vi "DriveModuleControl_TravTuneKa.vi"(8 "error in":errorcluster, 9 "Actual State":T1={"Speed"=0.0, "Angle"={"VALUE"=0.0, "COS"=1.0, "SIN"=0.0}} {"Angle"."SIN" format="%13.4f"; "Angle"."COS" format="%13.4f"; "Angle"."VALUE" format="%13.4f"}, 10 "Desired State":T1={"Speed"=0.0, "Angle"={"VALUE"=0.0, "COS"=1.0, "SIN"=0.0}} {"Angle"."SIN" format="%13.4f"; "Angle"."COS" format="%13.4f"; "Angle"."VALUE" format="%13.4f"}, 11 "ModualNamePrefix":i32) -> (0 "error out":errorcluster)   [LabVIEW 2023]
uses:
  <vilib>/Rock Robotics/WPI/ThirdParty/JAS_Junk/TrajLib/TypeDef/SWERVE_DRIVE_MODULE_STATE.ctl
  <vilib>/Rock Robotics/WPI/ThirdParty/JAS_Junk/TrajLib/TypeDef/ROTATION2D.ctl
  <vilib>/Rock Robotics/WPI/ThirdParty/JAS_Junk/TrajLib/Rotation2d_Minus.vi
  <vilib>/Rock Robotics/WPI/ThirdParty/JAS_Junk/TrajLib/Rotation2d_GetRadians.vi
  <vilib>/Rock Robotics/WPI/ThirdParty/JAS_Junk/TrajLib/SwerveModuleState_New.vi
  <vilib>/Rock Robotics/WPI/ThirdParty/JAS_Junk/TrajLib/Rotation2d_RotateBy.vi
  <vilib>/Rock Robotics/WPI/ThirdParty/JAS_Junk/TrajLib/Rotation2d_CreateAngle.vi
  <vilib>/Rock Robotics/WPI/ThirdParty/JAS_Junk/TrajLib/SimpleMotorFF_Calculate.vi
  <vilib>/Rock Robotics/WPI/ThirdParty/JAS_Junk/TrajLib/PIDController_AtSetpoint.vi
  <vilib>/Rock Robotics/WPI/ThirdParty/JAS_Junk/TrajLib/PIDController_SetPIDF.vi
  <vilib>/Rock Robotics/WPI/ThirdParty/JAS_Junk/TrajLib/PIDController_SetDerivativeFilter.vi
  <vilib>/Rock Robotics/WPI/ThirdParty/JAS_Junk/TrajLib/PIDController_SetIntegratorRange.vi
  <vilib>/Rock Robotics/WPI/ThirdParty/JAS_Junk/TrajLib/PIDController_SetTolerancePandV.vi
  <vilib>/Rock Robotics/WPI/ThirdParty/JAS_Junk/TrajLib/PIDController_DisableContinousInput.vi
  <vilib>/Rock Robotics/WPI/ThirdParty/JAS_Junk/TrajLib/PIDController_EnableContinousInput.vi
  <vilib>/Rock Robotics/WPI/ThirdParty/JAS_Junk/TrajLib/PIDController_Reset.vi
  <vilib>/Rock Robotics/WPI/ThirdParty/JAS_Junk/TrajLib/PIDController_New.vi
  <vilib>/Rock Robotics/WPI/ThirdParty/JAS_Junk/TrajLib/PIDController_SetOutputLimits.vi
  <vilib>/Rock Robotics/WPI/ThirdParty/JAS_Junk/TrajLib/VI/PIDController_SetIntegratorZone.vi
  <vilib>/Rock Robotics/WPI/ThirdParty/JAS_Junk/TrajLib/Rotation2d_UnaryMinus.vi
  <vilib>/Rock Robotics/WPI/ThirdParty/JAS_Junk/TrajLib/Rotation2d_CreateXY.vi
  <vilib>/Rock Robotics/WPI/ThirdParty/JAS_Junk/TrajLib/PIDController_NewPeriod.vi
  <vilib>/Rock Robotics/WPI/ThirdParty/JAS_Junk/TrajLib/Util_CalcDist.vi
  <vilib>/Rock Robotics/SystemInterfaces/NetworkCommunication/NetComm_UsageReport_report.vi
  DriveGlobal.vi
  <vilib>/Rock Robotics/WPI/ThirdParty/Phoenix6/Phoenix6_Device_RefNumRegistryGet.vi
  <vilib>/Rock Robotics/WPI/MotorControl/WPI_MotorControlRefNum Registry Get.vi
  <vilib>/Rock Robotics/Network Tables/NT Write Number.vi
  <vilib>/Rock Robotics/WPI/ThirdParty/JAS_Junk/TrajLib/Globals/Util_LibraryGlobals.vi
  <vilib>/Rock Robotics/WPI/ThirdParty/JAS_Junk/TrajLib/PIDController_AdvCalculate_FF_Sp_Pv.vi
  DriveTuningGlobals.vi
  <vilib>/Rock Robotics/Network Tables/NT Write Boolean.vi
  <vilib>/Rock Robotics/WPI/ThirdParty/JAS_Junk/TrajLib/Trajectory_Library.lvlib
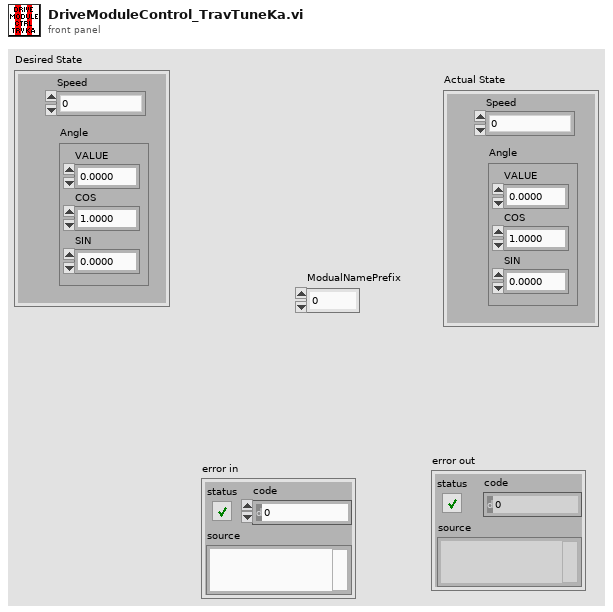
[diagram p1: front panel]
types:
  T1 = typedef "Trajectory_Library.lvlib/SWERVE_DRIVE_MODULE_STATE.ctl" = cluster{"Speed":dbl, "Angle":T2}
  T2 = typedef "Trajectory_Library.lvlib/ROTATION2D.ctl" = cluster{"VALUE":dbl, "COS":dbl, "SIN":dbl}
  T3 = typedef "WPI_MotorControlDeviceRef.ctl" = cluster{"DeviceStatus":errorcluster, "Type":T4, "PWM":cluster{"PWM Channel":T5, "DeadBand":T6}, "CAN":cluster{"Device Number":u8, "SetOutput VI Ref":variant, "GetOutput VI Ref":variant, "Enable VI Ref":variant, "Disable VI Ref":variant, "Data":variant}, "Invert":bool, "DIO PWM":cluster{"PWM \"Enable\" Channel":T5, "DIOChannel":T7, "PWM Rate":dbl}}
  T4 = typedef "WPI_MotorControlType.ctl" = enum16{"PWM", "CAN", "DIO PWM"}
  T5 = typedef "FPGA_DIOPWMChannel.ctl" = enum8{"PWM 0", "PWM 1", "PWM 2", "PWM 3", "PWM 4", "PWM 5", "PWM 6", "PWM 7", "PWM 8", "PWM 9", "PWM MXP 0", "PWM MXP 1", "PWM MXP 2", "PWM MXP 3", "PWM MXP 4", "PWM MXP 5", "PWM MXP 6", "PWM MXP 7", "PWM MXP 8", "PWM MXP 9", "Invalid"}
  T6 = typedef "WPI_PWMDeadband.ctl" = cluster{"Name":string, "maxPositivePwm":i32, "minPositivePwm":i32, "centerPwm":i32, "maxNegativePwm":i32, "minNegativePwm":i32, "angularRange":u16}
  T7 = typedef "FPGA_DIOChannel.ctl" = enum8{"DIO 0", "DIO 1", "DIO 2", "DIO 3", "DIO 4", "DIO 5", "DIO 6", "DIO 7", "DIO 8", "DIO 9", "DIO MXP 0", "DIO MXP 1", "DIO MXP 2", "DIO MXP 3", "DIO MXP 4", "DIO MXP 5", "DIO MXP 6", "DIO MXP 7", "DIO MXP 8", "DIO MXP 9", "DIO MXP 10", "DIO MXP 11", "DIO MXP 12", "DIO MXP 13", "DIO MXP 14", "DIO MXP 15", "SPI Port CS1", "SPI Port CS2", "SPI Port CS3", "SPI Port MISO", "SPI Port MOSI", "Invalid"}
  T8 = typedef "Trajectory_Library.lvlib/SIMPLE_MOTOR_FF.ctl" = cluster{"Ks":dbl, "Kv":dbl, "Ka":dbl, "KnInv":dbl}
  T9 = typedef "Trajectory_Library.lvlib/PID_ADV_LIMITS.ctl" = cluster{"MaxInput":dbl, "MinInput":dbl, "Continuous":bool, "MaxOutput":dbl, "MinOutput":dbl}
  T10 = typedef "Trajectory_Library.lvlib/PID_ADV_TUNING.ctl" = cluster{"Kf":dbl, "Kp":dbl, "Ki":dbl, "Kd":dbl, "MaximumIntegral":dbl, "MinimumIntegral":dbl, "Filter Derivative":bool, "IntegralZone":dbl}
  T11 = typedef "Trajectory_Library.lvlib/SIMPLE_MOTOR_FF_KA_TUNE_PARAMS.ctl" = cluster{"Max SP":dbl, "Min Eval SP":dbl, "Max Eval SP":dbl, "Ramp Rate":dbl}
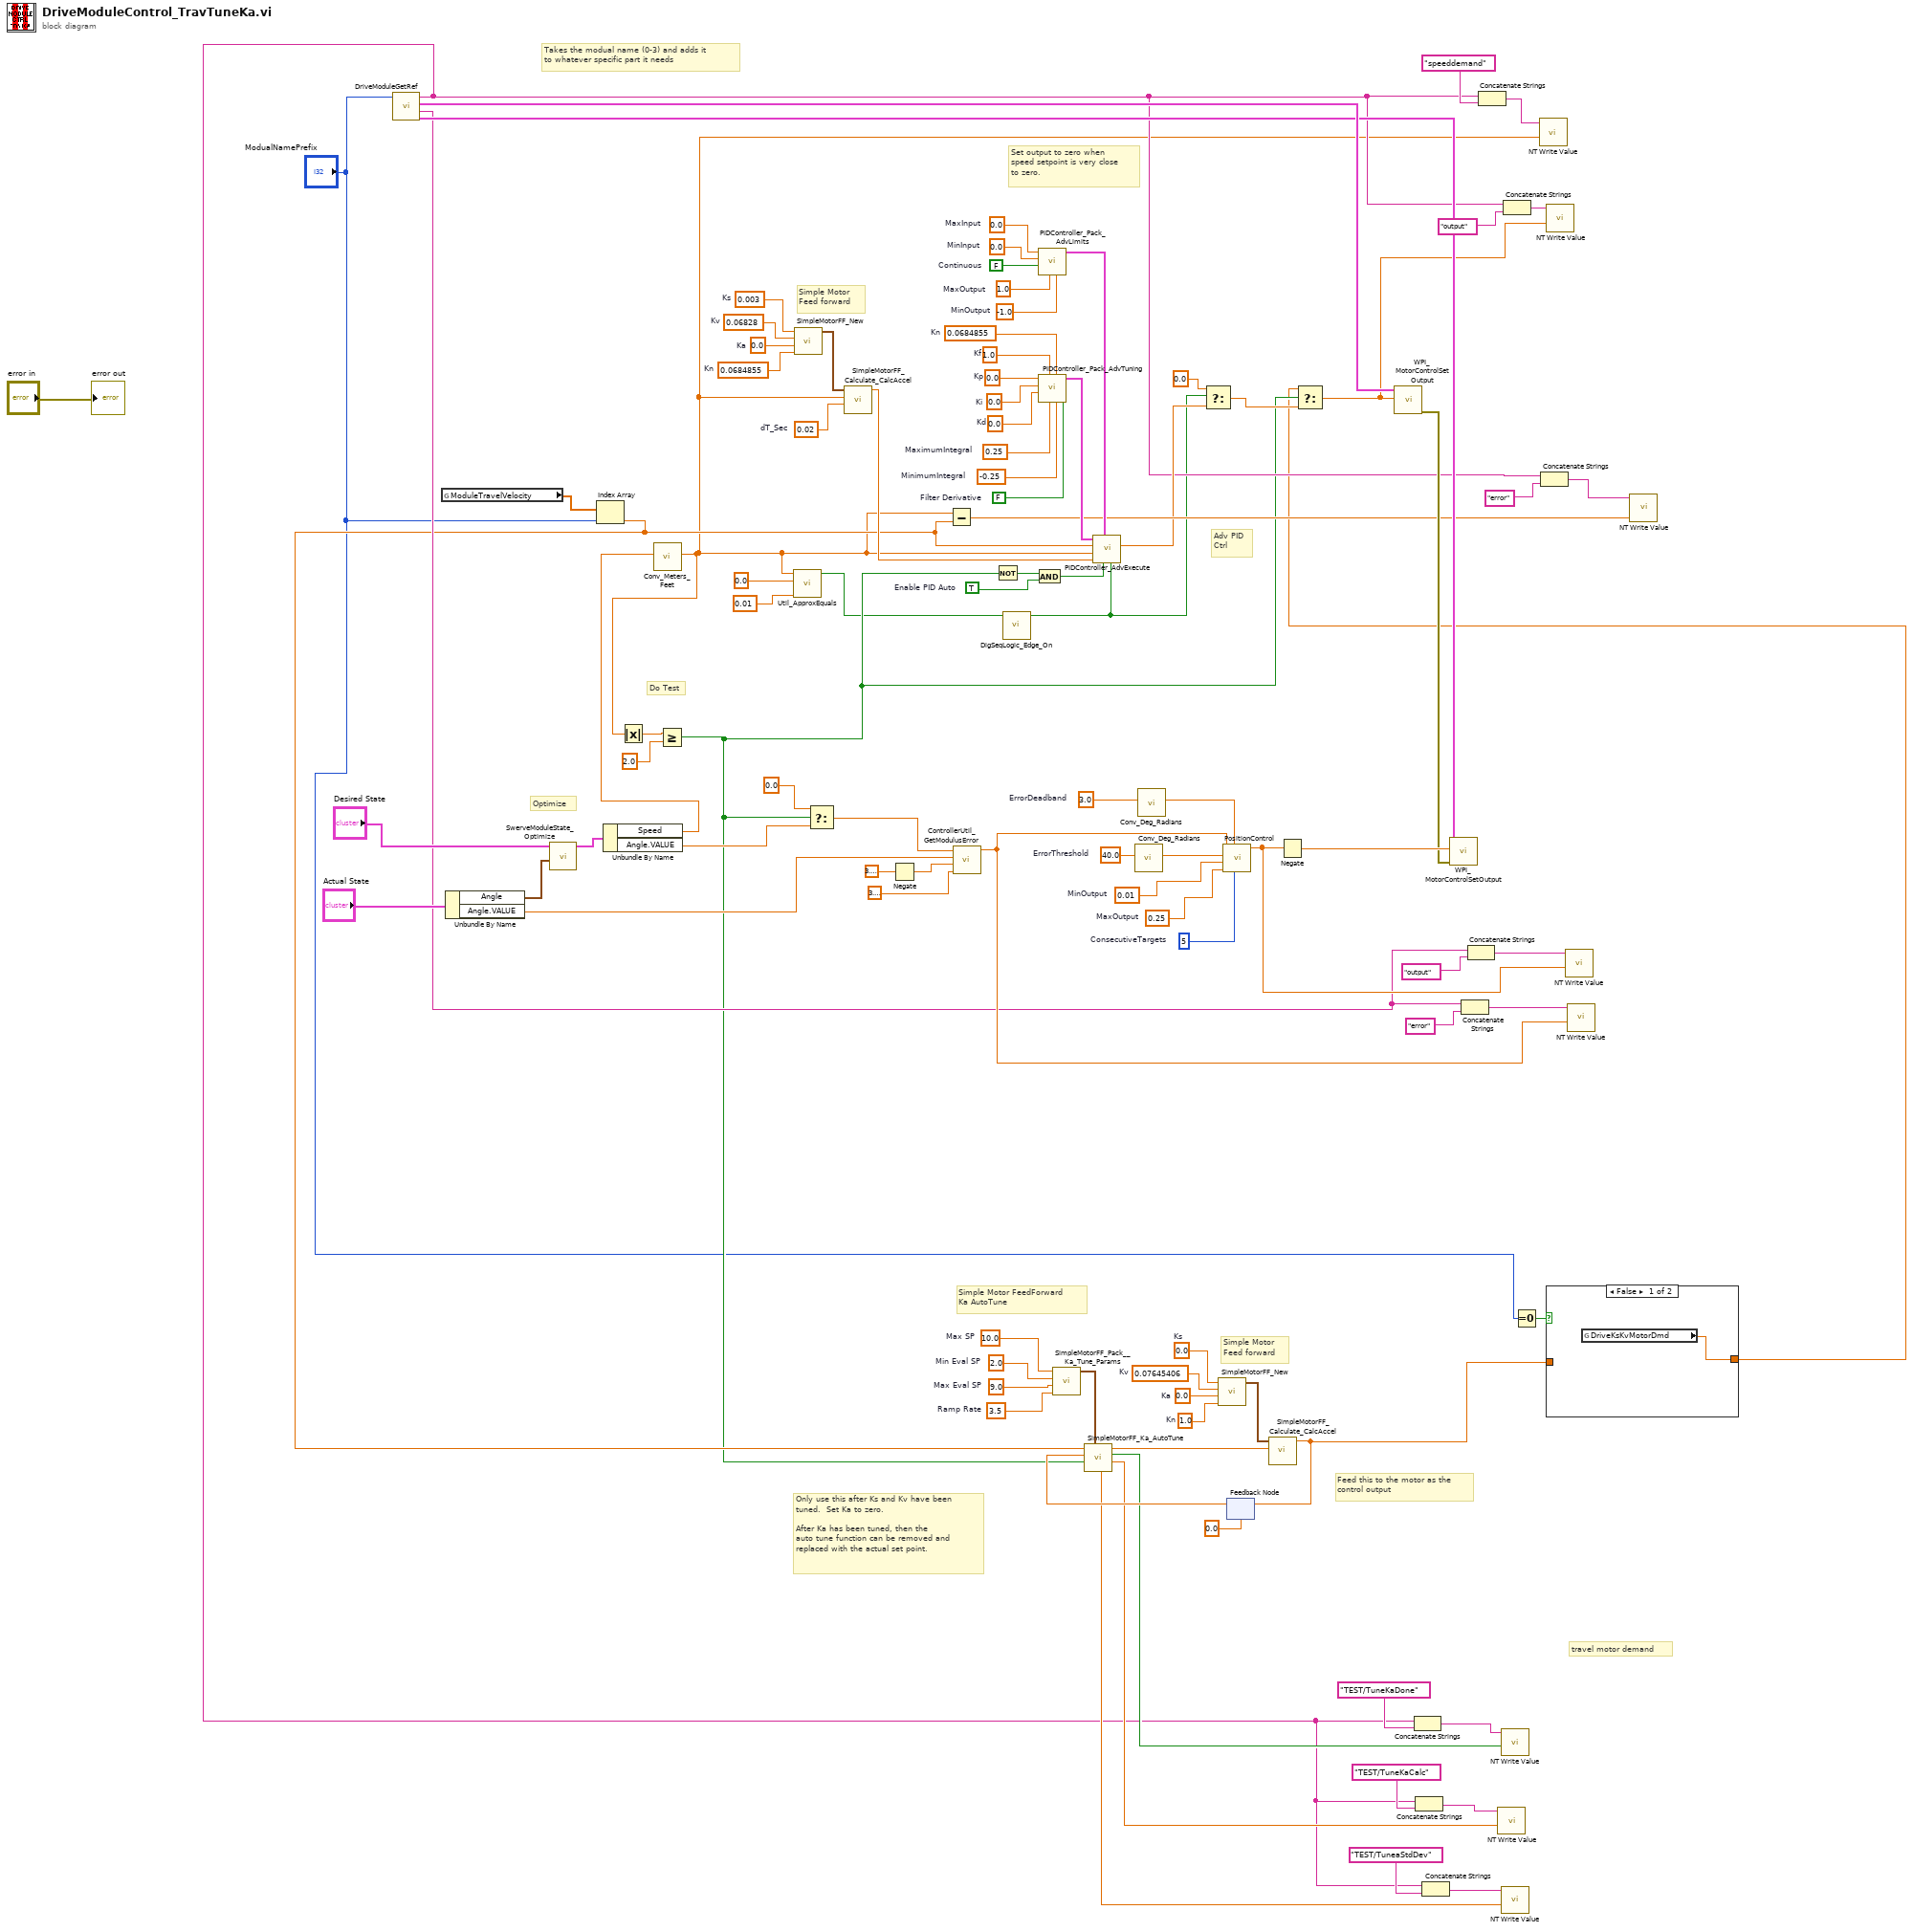
[diagram p0: block diagram]
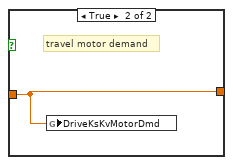
[diagram p2: hidden frame]
diagram:
  w29 = 1.0  # Kn
  w27 = 0.0  # Ks
  w26 = 0.07645406  # Kv
  w25 = 0.0  # Ka
  w24 = 10.0  # Max SP
  w23 = 2.0  # Min Eval SP
  w22 = 9.0  # Max Eval SP
  w21 = 3.5  # Ramp Rate
  w43 = TRUE  # Enable PID Auto
  w52 = 0.0684855  # Kn
  w68 = 0.0  # Kp
  w67 = 0.0  # Ki
  w66 = 0.0  # Kd
  w65 = 1.0  # Kf
  w64 = 0.25  # MaximumIntegral
  w63 = -0.25  # MinimumIntegral
  w62 = FALSE  # Filter Derivative
  w60 = 0.0  # MinInput
  w59 = FALSE  # Continuous
  w58 = 1.0  # MaxOutput
  w61 = -1.0  # MinOutput
  w57 = 0.0  # MaxInput
  w77 = 0.0684855  # Kn
  w76 = 0.02  # dT_Sec
  w74 = 0.003  # Ks
  w73 = 0.06828  # Kv
  w72 = 0.0  # Ka
  w87 = 5  # ConsecutiveTargets
  w84 = 0.25  # MaxOutput
  w88 = 0.01  # MinOutput
  w81 = 40.0  # ErrorThreshold
  w83 = 3.0  # ErrorDeadband
  # "Only use this after Ks and Kv have been\ntuned.  Set Ka to zero.\n\nAfter Ka has been tuned, then the \nauto tune function can be removed and\nreplaced with the actual set point."
  # "Feed this to the motor as the\ncontrol output"
  # "Simple Motor\nFeed forward"
  # "Simple Motor FeedForward\nKa AutoTune"
  # "travel motor demand"
  # "Do Test"
  # "Optimize"
  # "Set output to zero when\nspeed setpoint is very close\nto zero."
  # "Adv PID\nCtrl"
  # "Simple Motor\nFeed forward"
  # "Takes the modual name (0-3) and adds it \nto whatever specific part it needs"
  n1 = call "DriveModuleGetRef.vi"("ModualNamePrefix"="ModualNamePrefix") -> ("SpinMot"=w69:T3, "SpinStr"=w48:string, "TravMot"=w70:T3, "TravStr"=w9:string)  [unwired: 5 in, 2 out]
  n2 = global read "DriveGlobal.vi" "ModuleTravelVelocity"() -> (w53:dbl[])
  n3 = Unbundle By Name("Actual State") -> ("Angle"=w94:T2, "Angle.VALUE"=w91:dbl)
  n4 = call <vilib>:"SwerveModuleState_Optimize.vi"("CurrentAngle"=w94, "Desired State"="Desired State") -> ("out SWERVE_DRIVE_MODULE_STATE"=w92:T1)  [unwired: 9 in]
  n5 = Index Array(array=w53, index="ModualNamePrefix") -> (element=w16:dbl)
  n6 = Unbundle By Name(w92) -> ("Speed"=w40:dbl, "Angle.VALUE"=w37:dbl)
  n7 = call <vilib>:"Conv_Meters_Feet.vi"("Meters"=w40) -> ("Feet"=w7:dbl)  [unwired: 10 in]
  n8 = Absolute Value(x=w7) -> (abs(x)=w39:dbl)
  n9 = Greater Or Equal?(x=w39, y=2.0) -> (x >= y?=w8:bool)
  n10 = call <vilib>:"Util_ApproxEquals.vi"("Tolerance"=0.01, "Value 2"=0.0, "Value 1"=w7) -> ("ApproxEquals"=w2:bool)  [unwired: 8 in]
  n11 = call <vilib>:"SimpleMotorFF_New.vi"("Kn"=w77, "Ka"=w72, "Kv"=w73, "Ks"=w74) -> ("SIMPLE_MOTOR_FF"=w75:T8)  [unwired: 7 in]
  n12 = Select(t=0.0, s=w8, f=w37) -> (s? t:f=w33:dbl)
  n13 = call <vilib>:"SimpleMotorFF_Calculate_CalcAccel.vi"("dT_Sec"=w76, "VelSp"=w7, "SIMPLE_MOTOR_FF"=w75) -> ("FeedForward"=w54:dbl)  [unwired: 8 in]
  n14 = Negate(x=3.141592653589793) -> (-x=w93:dbl)
  n15 = Subtract(x=w7, y=w16) -> (x-y=w49:dbl)
  n16 = call <vilib>:"ControllerUtil_GetModulusError.vi"("Maximum_Input"=3.141592653589793, "Minimum_Input"=w93, "Measurerment(PV)"=w91, "Reference(SP)"=w33) -> ("Error"=w85:dbl)  [unwired: 7 in]
  n17 = Not(x=w8) -> (.not. x?=w44:bool)
  n18 = call <vilib>:"DigSeqLogic_Edge_On.vi"("Input"=w2) -> ("On Edge"=w1:bool)  [unwired: 10 in]
  n19 = And(x=w44, y=w43) -> (x .and. y?=w45:bool)
  n20 = call <vilib>:"PIDController_Pack_AdvLimits.vi"("MinOutput"=w61, "MaxOutput"=w58, "Continuous"=w59, "MinInput"=w60, "MaxInput"=w57) -> ("Adv PID Limits"=w55:T9)  [unwired: 6 in]
  n21 = call <vilib>:"PIDController_Pack_AdvTuning.vi"("Filter Derivative"=w62, "MinimumIntegral"=w63, "Kn"=w52, "MaximumIntegral"=w64, "Kf"=w65, "Kd"=w66, "Ki"=w67, "Kp"=w68) -> ("Adv PID Tuning"=w56:T10)  [unwired: 3 in]
  n22 = call <vilib>:"SimpleMotorFF_Pack__Ka_Tune_Params.vi"("Ramp Rate"=w21, "Max Eval SP"=w22, "Min Eval SP"=w23, "Max SP"=w24) -> ("Packed Params"=w20:T11)  [unwired: 7 in]
  n23 = call <vilib>:"PIDController_AdvExecute.vi"("Reset"=w1, "Auto"=w45, "Adv PID Limits"=w55, "FF-FeedForward"=w54, "SP-SetPoint"=w7, "PV-Measurement"=w16, "Adv PID Tuning"=w56) -> ("CO-ControlOutput"=w42:dbl)  [unwired: 2 in, 2 out]
  n24 = call <vilib>:"Conv_Deg_Radians.vi"("Degress"=w81) -> ("Radians"=w80:dbl)  [unwired: 10 in]
  n25 = call <vilib>:"Conv_Deg_Radians.vi"("Degress"=w83) -> ("Radians"=w82:dbl)  [unwired: 10 in]
  n26 = Select(t=0.0, s=w1, f=w42) -> (s? t:f=w34:dbl)
  n27 = call <vilib>:"SimpleMotorFF_New.vi"("Kn"=w29, "Ka"=w25, "Kv"=w26, "Ks"=w27) -> ("SIMPLE_MOTOR_FF"=w28:T8)  [unwired: 7 in]
  n28 = call "PositionControl.vi"("ConsecutiveTargets"=w87, "ErrorDeadband"=w82, "MaxOutput"=w84, "MinOutput"=w88, "ErrorThreshold"=w80, "Error"=w85) -> ("OutputValue"=w79:dbl)  [unwired: 3 in, 2 out]
  n29 = feedback #1(0.0 ("FeedForward")) -> (w31:dbl)
  n30 = call <vilib>:"SimpleMotorFF_Ka_AutoTune.vi"("SimpleMotorFeedforward_KaTune_Pack"=w20, "Run Test"=w8, "CO Control Output"=w31, "PV ProcessVariable"=w16) -> ("Ka Calc"=w18:dbl, "Test Complete"=w19:bool, "SP Setpoint"=w30:dbl, "Ka StdDev"=w17:dbl)  [unwired: 1 in, 3 out]
  n31 = call <vilib>:"SimpleMotorFF_Calculate_CalcAccel.vi"("VelSp"=w30, "SIMPLE_MOTOR_FF"=w28) -> ("FeedForward"=w5:dbl)  [unwired: 9 in]
  n32 = feedback-in #1(w5) -> ()
  n33 = Negate(x=w79) -> (-x=w78:dbl)
  n34 = Concatenate Strings(w9, "TEST/TuneKaDone" ("name")) -> (w12:string)
  n35 = Concatenate Strings(w9, "TEST/TuneKaCalc" ("name")) -> (w11:string)
  n36 = Concatenate Strings(w9, "TEST/TuneaStdDev" ("name")) -> (w10:string)
  n37 = Concatenate Strings(w48, "error" ("refnum name")) -> (w98:string)
  n38 = Concatenate Strings(w48, "output" ("refnum name")) -> (w86:string)
  n39 = Concatenate Strings(w9, "speeddemand" ("refnum name")) -> (w102:string)
  n40 = call-poly <vilib>:"NT Write Value.vi"("value"=w18, "name"=w11) -> ()  [unwired: 9 in, 1 out]
  n41 = call-poly <vilib>:"NT Write Value.vi"("value"=w19, "name"=w12) -> ()  [unwired: 9 in, 1 out]
  n42 = call-poly <vilib>:"NT Write Value.vi"("value"=w17, "name"=w10) -> ()  [unwired: 9 in, 1 out]
  n43 = Concatenate Strings(w9, "output" ("refnum name")) -> (w100:string)
  n44 = Equal To 0?(x="ModualNamePrefix") -> (x = 0?=w6:bool)
  n45 = call-poly <vilib>:"NT Write Value.vi"("value"=w7, "name"=w102) -> ()  [unwired: 9 in, 1 out]
  n46 = Concatenate Strings(w9, "error" ("refnum name")) -> (w50:string)
  n47 = case shown="False" w6 {
    tunnel: w5 -> [_ w106]
    tunnel: [w105 w106] -> w4
    frame False {
      n48 = global read "DriveTuningGlobals.vi" "DriveKsKvMotorDmd"() -> (w105:dbl)
    }
    frame True {
      # "travel motor demand"
      n49 = global write "DriveTuningGlobals.vi" "DriveKsKvMotorDmd"(w106) -> ()
    }
  }
  n50 = Select(t=w4, s=w8, f=w34) -> (s? t:f=w35:dbl)
  n51 = call <vilib>:"WPI_MotorControlSetOutput.vi"("Output"=w35, "MotorControlDevRef"=w70) -> ("error out"=w71:errorcluster)  [unwired: 7 in, 2 out]
  n52 = call <vilib>:"WPI_MotorControlSetOutput.vi"("error in (no error)"=w71, "Output"=w78, "MotorControlDevRef"=w69) -> ()  [unwired: 6 in, 3 out]
  n53 = call-poly <vilib>:"NT Write Value.vi"("value"=w35, "name"=w100) -> ()  [unwired: 9 in, 1 out]
  n54 = call-poly <vilib>:"NT Write Value.vi"("value"=w79, "name"=w86) -> ()  [unwired: 9 in, 1 out]
  n55 = call-poly <vilib>:"NT Write Value.vi"("value"=w85, "name"=w98) -> ()  [unwired: 9 in, 1 out]
  n56 = call-poly <vilib>:"NT Write Value.vi"("value"=w49, "name"=w50) -> ()  [unwired: 9 in, 1 out]
  "error out" <- "error in"
